vi "APC_9049_float2u16.vi"(1 "min":sgl[](array[numeric]), 2 "holding register values":sgl[](array[numeric]), 3 "max":sgl[](array[numeric])) -> (0 "uint16 array":u16[](array[numeric]))   [LabVIEW 2020]
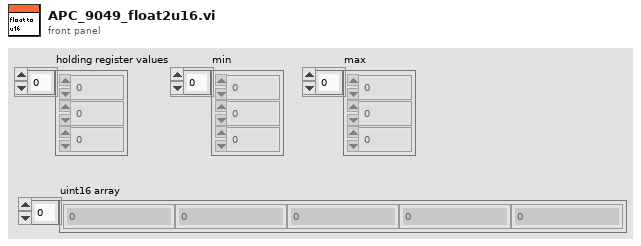
[diagram p1: front panel]
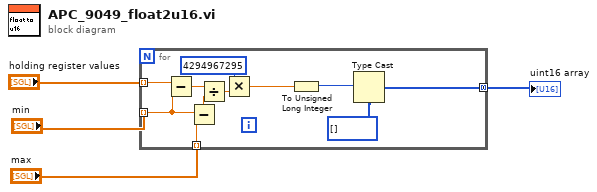
[diagram p0: block diagram]
diagram:
  n1 = for {
    tunnel: "holding register values" -> [w15] mode=indexing
    tunnel: "min" -> [w10] mode=indexing
    tunnel: "max" -> [w11] mode=indexing
    tunnel: [w5] -> w1 mode=concatenating
    n2 = Subtract(x=w15, y=w10) -> (x-y=w14:sgl)
    n3 = Subtract(x=w11, y=w10) -> (x-y=w9:sgl)
    n4 = Divide(x=w14, y=w9) -> (x/y=w13:sgl)
    n5 = Multiply(x=u32 4294967295, y=w13) -> (x*y=w8:sgl)
    n6 = To Unsigned Long Integer(number=w8) -> (unsigned 32bit integer=w6:u32)
    n7 = Type Cast(type=u16[] [] ("register values 2"), x=w6) -> (*(type *) &x=w5:u16[])
  }
  "uint16 array" <- w1
